vi "Callback_WebMessage.vi"(4 "WebResourceResponseData":refnum<user-event>, 5 "Event Data":cluster{"sender":refnum<k24>, "e":refnum<k24>}, 6 "Control Ref":refnum<k24>, 7 "Event Common Data":T1) -> ()   [LabVIEW 2020, in "DP_WebView.lvclass"]
uses:
  DP_WebView.lvclass
  C:/Projects/DependencyViewer/DependencyViewer/DP_WebView_class/data/Microsoft.Web.WebView2.Core.dll
  data/Microsoft.Web.WebView2.Core.dll
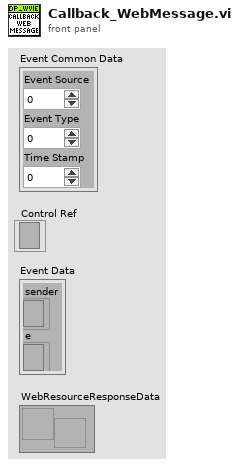
[diagram p1: front panel]
types:
  T1 = cluster{"Event Source":i32, "Event Type":u32, "Time Stamp":u32}
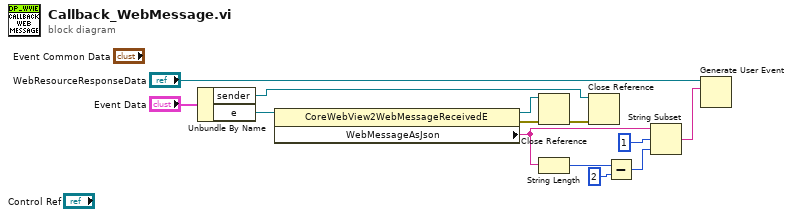
[diagram p0: block diagram]
diagram:
  n1 = Unbundle By Name("Event Data") -> ("sender"=w7:refnum<k24>, "e"=w11:refnum<k24>)
  n2 = property class="CoreWebView2WebMessageReceivedE"(reference=w11) -> (reference out=w9:refnum<k24>, error out=w10:errorcluster, "WebMessageAsJson"=w2:string)  [unwired: 1 in]
  n3 = Close Reference(reference=w9, error in (no error)=w10) -> (error out=w8:errorcluster)
  n4 = String Length(string=w2) -> (length=w6:i32)
  n5 = Close Reference(reference=w7, error in (no error)=w8) -> ()  [unwired: 1 out]
  n6 = Subtract(x=w6, y=2) -> (x-y=w3:i32)
  n7 = String Subset(string=w2, offset (0)=1, length (rest)=w3) -> (substring=w1:string)
  n8 = Generate User Event(user event="WebResourceResponseData", event data cluster=w1) -> ()  [unwired: 2 in, 2 out]
